vi "Filter Tree.vi"(7 "Headers":string[](array[string]), 8 "error in":errorcluster, 9 "Tags map":refnum<vi>, 10 "Frames":refnum<vi>, 11 "Filter":refnum<vi>) -> (0 "error out":errorcluster)   [LabVIEW 2025, in "CAN-LIN Raw Bus Capture UI.lvlib"]
uses:
  CAN-LIN Raw Bus Capture UI.lvlib
  <vilib>/Utility/error.llb/whitespace.ctl
  Table_Filtering/Table_Filtering.lvlib
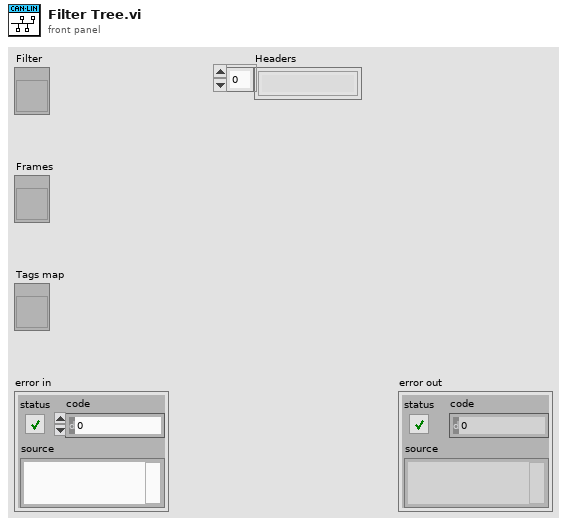
[diagram p1: front panel]
types:
  T1 = typedef "whitespace.ctl" = u16
  T2 = cluster{"FIELD":string, "OPERATOR":string, "VALUE":string}[]
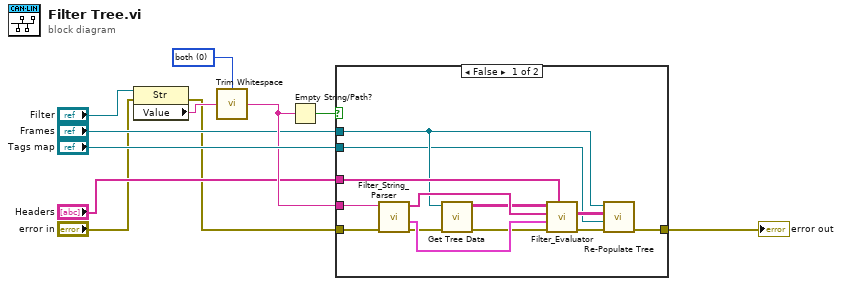
[diagram p0: block diagram]
diagram:
  w6 = T1 0 items=["both", "start of string", "end of string"] ("location (both)")
  n1 = property class="Str"(reference="Filter", error in="error in") -> (error out=w1:errorcluster, "Value"=w11:string)  [unwired: 1 out]
  n2 = call <vilib>:"Trim Whitespace.vi"("string"=w11, "location (both)"=w6) -> ("trimmed string"=w7:string)
  n3 = Empty String/Path?(string/path=w7) -> (empty?=w8:bool)
  n4 = case shown="False" w8 {
    tunnel: w1 -> [w24 w25]
    tunnel: "Headers" -> [w21 _]
    tunnel: "Frames" -> [w15 _]
    tunnel: [w14 w25] -> w5
    tunnel: w7 -> [w13 _]
    tunnel: "Tags map" -> [w12 _]
    frame False {
      n5 = call "Filter_String_Parser.vi"("error in"=w24, "Filter String"=w13) -> ("error constant"=w18:errorcluster, "Comparators"=w23:T2, "Boolean Connectors"=w22:string[])  [unwired: 7 in]
      n6 = call "Get Tree Data.vi"("error in"=w18, "Tree ref"=w15) -> ("error out"=w19:errorcluster, "Array"=w20:string[][])  [unwired: 8 in]
      n7 = call "Filter_Evaluator.vi"("Headers"=w21, "Error"=w19, "Comparators"=w23, "Boolean Connectors"=w22, "Prefiltered Data"=w20) -> ("Error Out"=w16:errorcluster, "Filtered Array"=w17:string[][])  [unwired: 4 in, 1 out]
      n8 = call "Re-Populate Tree.vi"("error in"=w16, "Tags map"=w12, "Data in"=w17, "TreeControl in"=w15) -> ("error out"=w14:errorcluster)  [unwired: 7 in]
    }
    frame True {
    }
  }
  "error out" <- w5
